vi "Read 2d data.vi"(5 "Col Param Path":string, 7 "Row Param Path":string, 8 "error in (no error)":errorcluster, 10 "Parameter Path":string, 11 ".NET Refnum in":T1) -> (0 "error out":errorcluster, 3 "TBL2D":cluster{"X":sgl[], "Y":sgl[], "Z":sgl[][]})   [LabVIEW 2011]
uses:
  <vilib>/NI Veristand/Execution/ModelManager/ModelManagerAPI.ctl
  NationalInstruments.VeriStand.ClientAPI
  <vilib>/NI Veristand/Execution/ModelManager/NI VeriStand - Get Parameter 2D Array Values.vi
  <vilib>/NI Veristand/Execution/ModelManager/NI_VS ModelManager ExecutionAPI.lvlib
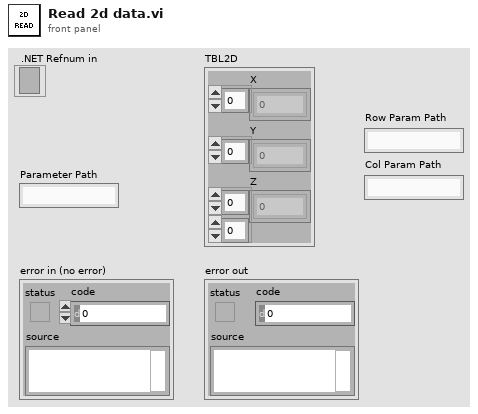
[diagram p1: front panel]
types:
  T1 = typedef "NI_VS ModelManager ExecutionAPI.lvlib/ModelManagerAPI.ctl" = refnum<k24>
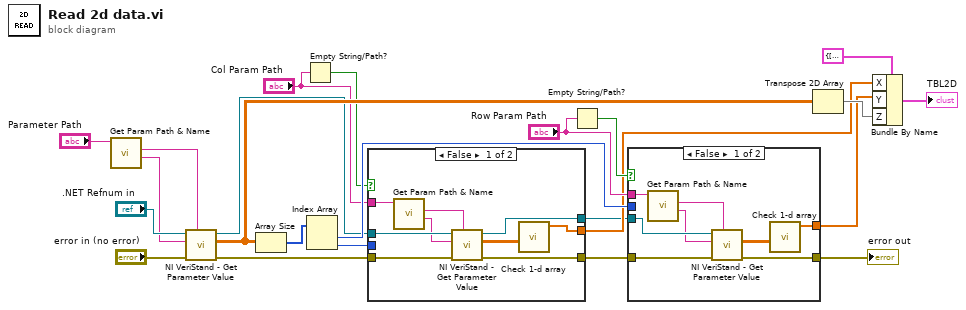
[diagram p0: block diagram]
diagram:
  n1 = call "Get Param Path & Name.vi"("Path"="Parameter Path") -> ("Parameter Path"=w12:string, "Controller name"=w13:string)  [unwired: 8 in, 1 out]
  n2 = call-poly <vilib>:"NI VeriStand - Get Parameter Value.vi"("Target"=w13, "error in (no error)"="error in (no error)", "Parameter"=w12, "ModelManager in"=".NET Refnum in") -> ("error out"=w8:errorcluster, "Values"=w17:dbl[][], "ModelManager out"=w5:T1)  [unwired: 5 in]
  n3 = Array Size(array=w17) -> (size(s)=w18:i32[])
  n4 = Empty String/Path?(string/path="Col Param Path") -> (empty?=w1:bool)
  n5 = Index Array(array=w18) -> (element #1=w23:i32, element #2=w7:i32)  [unwired: 2 in]
  n6 = case shown="False" w1 {
    tunnel: w7 -> [_ w36]
    tunnel: [w26 w35] -> w6
    tunnel: "Col Param Path" -> [w32 _]
    tunnel: w8 -> [w31 w34]
    tunnel: w5 -> [w30 w33]
    tunnel: [w25 w34] -> w3
    tunnel: [w24 w33] -> w4
    frame False {
      n7 = call "Get Param Path & Name.vi"("Path"=w32) -> ("Parameter Path"=w29:string, "Controller name"=w28:string)  [unwired: 8 in, 1 out]
      n8 = call-poly <vilib>:"NI VeriStand - Get Parameter Value.vi"("Target"=w28, "error in (no error)"=w31, "Parameter"=w29, "ModelManager in"=w30) -> ("error out"=w25:errorcluster, "Values"=w27:dbl[][], "ModelManager out"=w24:T1)  [unwired: 5 in]
      n9 = call "Check 1-d array.vi"("Array"=w27) -> ("Array 2"=w26:dbl[])  [unwired: 10 in]
    }
    frame True {
      n10 = for {
        N: w36 -> [_]
        tunnel: [w37] -> w35 mode=indexing
        i -> [w37]
      }
    }
  }
  n11 = Empty String/Path?(string/path="Row Param Path") -> (empty?=w11:bool)
  n12 = case shown="False" w11 {
    tunnel: w23 -> [_ w48]
    tunnel: [w39 w47] -> w21
    tunnel: "Row Param Path" -> [w45 _]
    tunnel: w3 -> [w44 w46]
    tunnel: w4 -> [w43 _]
    tunnel: [w38 w46] -> w9
    frame False {
      n13 = call "Get Param Path & Name.vi"("Path"=w45) -> ("Parameter Path"=w42:string, "Controller name"=w41:string)  [unwired: 8 in, 1 out]
      n14 = call-poly <vilib>:"NI VeriStand - Get Parameter Value.vi"("Target"=w41, "error in (no error)"=w44, "Parameter"=w42, "ModelManager in"=w43) -> ("error out"=w38:errorcluster, "Values"=w40:dbl[][])  [unwired: 5 in, 1 out]
      n15 = call "Check 1-d array.vi"("Array"=w40) -> ("Array 2"=w39:dbl[])  [unwired: 10 in]
    }
    frame True {
      n16 = for {
        N: w48 -> [_]
        tunnel: [w49] -> w47 mode=indexing
        i -> [w49]
      }
    }
  }
  "error out" <- w9
  n17 = Transpose 2D Array(2D array=w17) -> (transposed array=w22:dbl[][])
  n18 = Bundle By Name(cluster=cluster{"X":sgl[], "Y":sgl[], "Z":sgl[][]} {"X"=[], "Y"=[], "Z"=[]} ("TBL2D"), "X"=w6, "Y"=w21, "Z"=w22) -> (→"TBL2D":cluster{"X":sgl[], "Y":sgl[], "Z":sgl[][]})
